vi "OverlayArcBoundingBox.vi"(4 "GroupName":string, 6 "Color":u32(colorbox)=16711680, 7 "Angles":T1 {"End Angle (degrees)" format="%.2f"; "Start Angle (degrees)" format="%.2f"}, 8 "error in":errorcluster, 9 "Drawing Mode (Frame)":T3, 10 "BondingBox":T2, 11 "Image Reference In":T4) -> (0 "error out":errorcluster, 3 "Image Reference Out":T4)   [LabVIEW 2020, in "OpenLvVision_Overlays.lvlib"]
doc: "Overlay a arc on top of an image.\nDraws it by the given bounding box coordinates."
uses:
  OpenLvVision_Overlays.lvlib
  <vilib>/OpenLvVision/OpenLvVision_Image/Management/TypeDef/OLV Image.ctl
  <vilib>/OpenLvVision/OpenLvVision_Image/Management/OLV Management.lvlib
  TypeDefs/DrawingMode.ctl
  <vilib>/OpenLvVision/OpenLvVision_Image/DataAccess/TypeDef/OLV RectangleI32.ctl
  <vilib>/OpenLvVision/OpenLvVision_Image/DataAccess/OLV DataAccess.lvlib
  TypeDefs/Angles.ctl
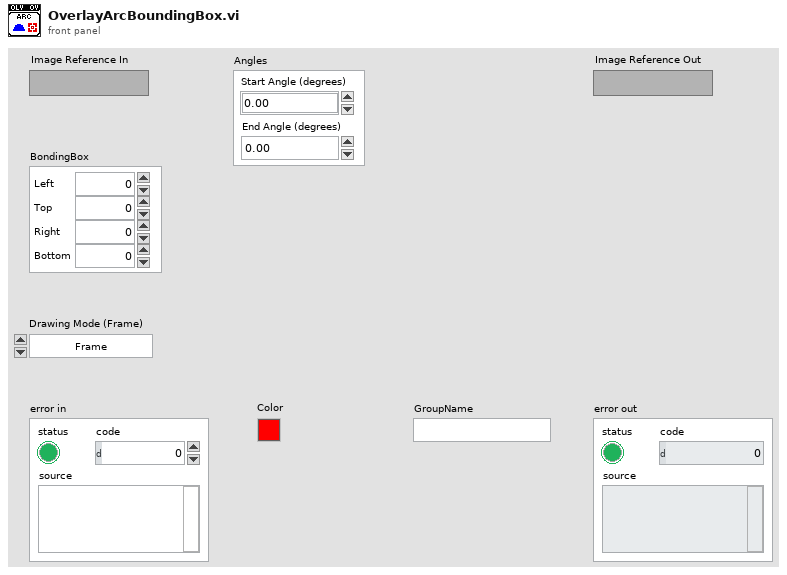
[diagram p1: front panel]
types:
  T1 = typedef "OpenLvVision_Overlays.lvlib/Angles.ctl" = cluster{"Start Angle (degrees)":dbl, "End Angle (degrees)":dbl}
  T2 = typedef "OLV OpenLvVision_Image.lvlib/OLV DataAccess.lvlib/OLV RectangleI32.ctl" = cluster{"Left":i32, "Top":i32, "Right":i32, "Bottom":i32}
  T3 = typedef "OpenLvVision_Overlays.lvlib/DrawingMode.ctl" = enum16{"Frame", "Fill"}
  T4 = typedef "OLV OpenLvVision_Image.lvlib/OLV Management.lvlib/OLV Image.ctl" = refnum<image>
  T5 = typedef "IMAQ Image.ctl" = refnum<image>
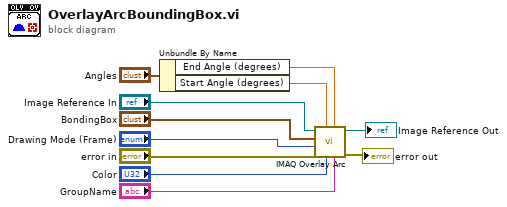
[diagram p0: block diagram]
diagram:
  n1 = Unbundle By Name("Angles") -> ("End Angle (degrees)"=w1:dbl, "Start Angle (degrees)"=w2:dbl)
  n2 = call "IMAQ Overlay Arc"("Group"="GroupName", "End Angle (degrees)"=w1, "Color"="Color", "Start Angle (degrees)"=w2, "error in (no error)"="error in", "Drawing Mode (Frame)"="Drawing Mode (Frame)", "Bounding Rectangle"="BondingBox", "Image"="Image Reference In") -> ("error out"=→"error out":errorcluster, "Image Out"=→"Image Reference Out":T5)  [unwired: 2 in]
